vi "dataFiltering(SubVI).vi"(0 "dataIN":dbl, 1 "shiftREG_in":dbl, 5 "Degree":i32, 6 "highRange_data":dbl, 8 "lowRange_data":dbl, 10 "highRange_avgData":dbl, 12 "lowRange_avgData":dbl, 13 "GivenValue":dbl) -> (11 "shiftREG_out":dbl, 14 "rawData":dbl, 15 "inRange_rawData":bool, 16 "exAvg_data":dbl, 17 "inRange_avgData":bool, 18 "diff_AvgRaw":dbl, 19 "lessThanGivenValue":bool)   [LabVIEW 2017]
panel:
  in  "iteration":dbl
  out "Waveform Chart":cluster{dbl, dbl}(graph)
  # "Low degree provides\ncloser fit between \nfiltered and raw data"
  # "*also degree\nof 0 gives\nan error"
  # "At some point I want\nto use this \"given value\"\nto determine degree\nof incoming data"
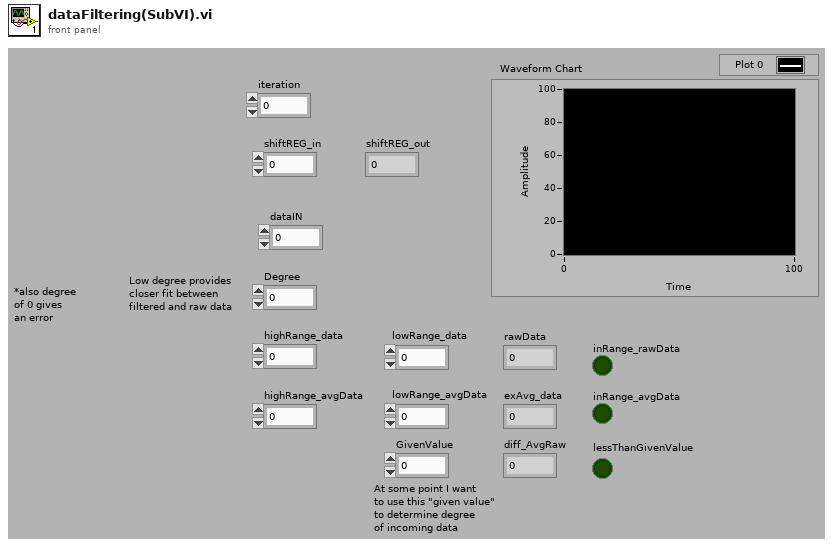
[diagram p1: front panel]
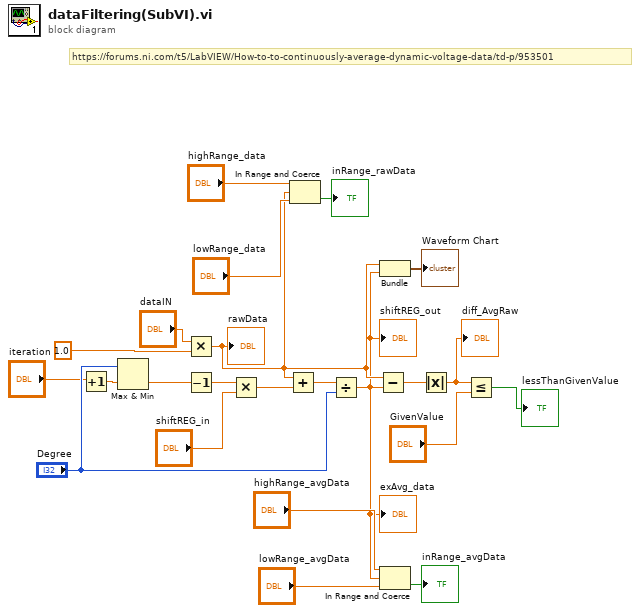
[diagram p0: block diagram]
diagram:
  # "https://forums.ni.com/t5/LabVIEW/How-to-to-continuously-average-dynamic-voltage-data/td-p/953501"
  n1 = Increment(x="iteration") -> (x+1=w20:dbl)
  n2 = Max & Min(x="Degree", y=w20) -> (min(x,y)=w19:dbl)  [unwired: 1 out]
  n3 = Multiply(x="dataIN", y=1.0) -> (x*y=w6:dbl)
  "rawData" <- w6
  n4 = Decrement(x=w19) -> (x-1=w23:dbl)
  n5 = Multiply(x=w23, y="shiftREG_in") -> (x*y=w21:dbl)
  n6 = Add(x=w6, y=w21) -> (x+y=w22:dbl)
  n7 = In Range and Coerce(upper limit="highRange_data", x=w6, lower limit="lowRange_data") -> (In Range?=→"inRange_rawData":bool)  [unwired: 1 out]
  n8 = Divide(x=w22, y="Degree") -> (x/y=w2:dbl)
  "exAvg_data" <- w2
  "shiftREG_out" <- w2
  n9 = Subtract(x=w6, y=w2) -> (x-y=w17:dbl)
  n10 = Bundle(w6, w2) -> (→"Waveform Chart":cluster{dbl, dbl})  [unwired: 1 in]
  n11 = In Range and Coerce(upper limit="highRange_avgData", x=w2, lower limit="lowRange_avgData") -> (In Range?=→"inRange_avgData":bool)  [unwired: 1 out]
  n12 = Absolute Value(x=w17) -> (abs(x)=w9:dbl)
  "diff_AvgRaw" <- w9
  n13 = Less Or Equal?(x=w9, y="GivenValue") -> (x <= y?=→"lessThanGivenValue":bool)
